vi "YOST 3 Space Loop.vi"() -> ()   [LabVIEW 2012]
uses:
  <vilib>/Platform/TimedLoop/XDataNode/XDataNode.xnode
  <vilib>/Platform/TimedLoop/XDataNode/nitl_modes.ctl
  <vilib>/Platform/TimedLoop/XDataNode/XDNodeRunTimeDep.lvlib
  <vilib>/Platform/TimedLoop/XDataNode/wakeup.ctl
  <vilib>/Platform/TimedLoop/XDataNode/timing_clust.ctl
  YOST 3 Space.lvlib
  <vilib>/robotics/Controls/Compass Indicator/Compass Indicator.xctl
  <vilib>/robotics/Controls/Attitude Indicator/Attitude Indicator.xctl
panel:
  out "LED Mode":i32
  out "IMU Data":T1
  in  "ID Query (True)":bool=TRUE
  out "Attitude Indicator":cluster{"Roll":dbl, "Pitch":dbl}(xcontrol)
  out "Compass Indicator":dbl(xcontrol)
  in  "error in":errorcluster
  out "error out":errorcluster
  in  "stop?":bool
  in  "Debug":bool
  in  "VISA resource name":refnum<visa-resource-name>
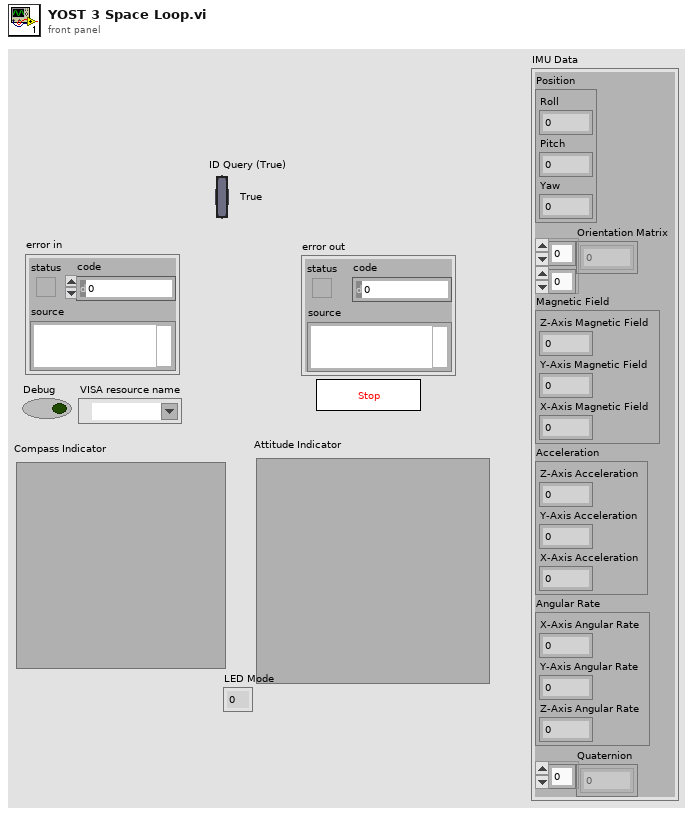
[diagram p1: front panel]
types:
  T1 = cluster{"Position":cluster{"Roll":dbl, "Pitch":dbl, "Yaw":dbl}, "Orientation Matrix":dbl[][], "Magnetic Field":cluster{"Z-Axis Magnetic Field":dbl, "Y-Axis Magnetic Field":dbl, "X-Axis Magnetic Field":dbl}, "Acceleration":cluster{"Z-Axis Acceleration":dbl, "Y-Axis Acceleration":dbl, "X-Axis Acceleration":dbl}, "Angular Rate":cluster{"X-Axis Angular Rate":dbl, "Y-Axis Angular Rate":dbl, "Z-Axis Angular Rate":dbl}, "Quaternion":dbl[]}
  T2 = typedef "XDNodeRunTimeDep.lvlib/timing_clust.ctl" = cluster{"Expected End [f-1]":u64, "Actual End [f-1]":u64, "Finished Late? [f-1]":bool, "Expected End [i-1]":u64, "Actual End [i-1]":u64, "Finished Late? [i-1]":bool, "Expected Start [i]":u64, "Actual Start [i]":u64, "Expected Start [f]":u64, "Actual Start [f]":u64, "Source Name":string, "Structure Name":string, "Period":i64, "Deadline":i64, "Offset":i64, "Start":i64, "Priority":i32, "Timeout":i32, "Mode":T3, "Wakeup Reason":T4, "Error":errorcluster, "Source Type":string, "Secondary Source Type":string, "Global End Time":u64, "Global Start Time":u64, "Frame Duration":u64, "Iteration Duration":u64, "Assigned CPU":i32, "I/O Scan Engine Mode":u32}
  T3 = typedef "XDNodeRunTimeDep.lvlib/nitl_modes.ctl" = enum32{"No Change", "Process missed periods, maintain original phase", "Discard missed periods, maintain original phase", "Process missed periods, ignore original phase", "Discard missed periods, ignore original phase"}
  T4 = typedef "XDNodeRunTimeDep.lvlib/wakeup.ctl" = enum32{"Normal", "Aborted", "Asynchronous wakeup", "Timing source error", "Timed loop error", "Timeout"}
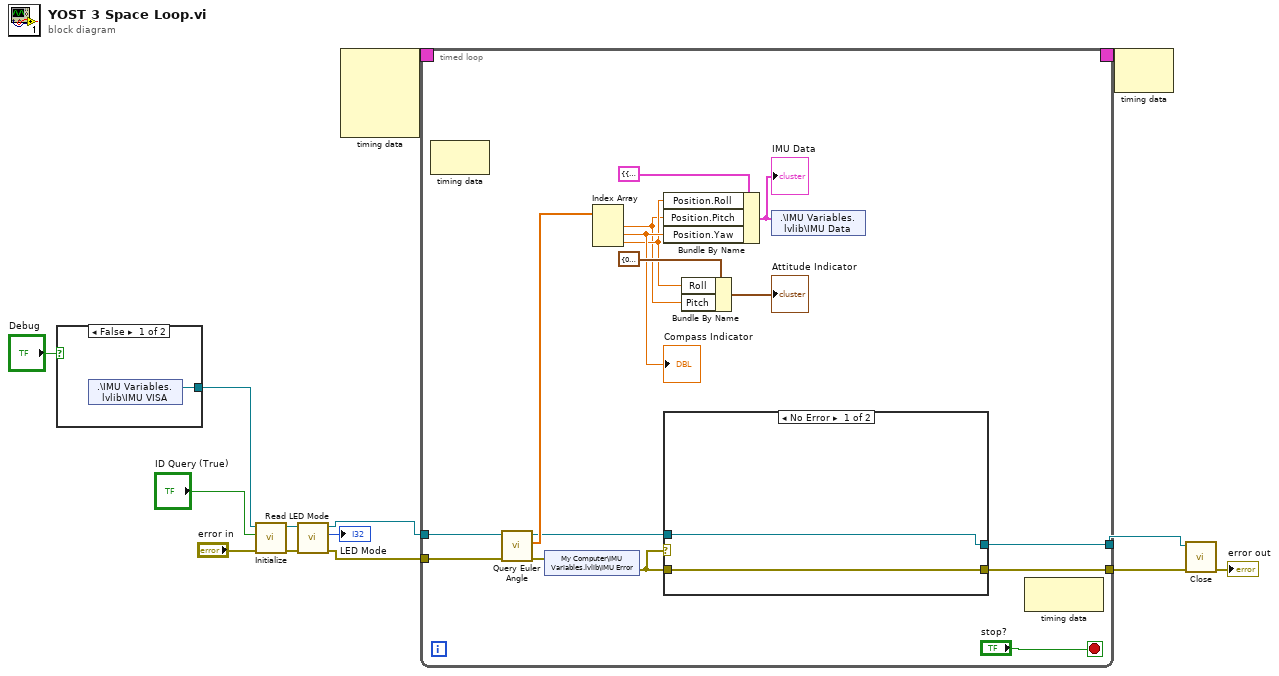
[diagram p0: block diagram]
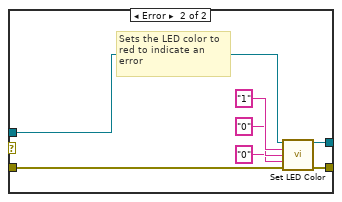
[diagram p2: hidden frame]
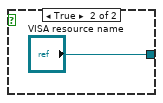
[diagram p3: hidden frame]
diagram:
  n1 = case shown="False" "Debug" {
    tunnel: [w15 "VISA resource name"] -> w10
    frame False {
      n2 = shared-variable ".\\IMU Variables.lvlib\\IMU VISA"() -> (w15:refnum<visa-resource-name>)  [unwired: 1 in, 1 out]
    }
    frame True {
    }
  }
  n3 = call "Initialize.vi"("error in (no error)"="error in", "ID Query (True)"="ID Query (True)", "VISA resource name"=w10) -> ("error out"=w6:errorcluster, "VISA resource name out"=w5:refnum<visa-resource-name>)  [unwired: 7 in]
  n4 = call "Read LED Mode.vi"("error in"=w6, "Session In"=w5) -> ("error out"=w7:errorcluster, "Mode"=→"LED Mode":i32, "Session Out"=w4:refnum<visa-resource-name>)  [unwired: 7 in]
  n5 = node-c288() -> (w13:T2)  [unwired: 4 in]
  n6 = timed-loop {
    timing: w13 -> [_]
    timing-out: [_] -> w12
    tunnel: [w17] -> w1
    tunnel: w4 -> [w22]
    tunnel: w7 -> [w21]
    tunnel: [w18] -> w2
    stop <- "stop?" stop-if-true
    n7 = node-c288() -> ()  [unwired: 1 in, 1 out]
    n8 = call "Query Euler Angle.vi"("error in"=w21, "Session In"=w22) -> ("error out"=w20:errorcluster, "Euler Angles"=w29:dbl[], "Session Out"=w19:refnum<visa-resource-name>)  [unwired: 7 in]
    n9 = shared-variable "My Computer\\IMU Variables.lvlib\\IMU Error"(w20) -> (error out=w23:errorcluster)  [unwired: 1 in]
    n10 = Index Array(array=w29) -> (element #1=w24:dbl, element #2=w26:dbl, element #3=w25:dbl)  [unwired: 3 in]
    "Compass Indicator" <- w26
    n11 = Bundle By Name(cluster=T1 {"Position"={"Roll"=0.0, "Pitch"=0.0, "Yaw"=0.0}, "Orientation Matrix"=[], "Magnetic Field"={"Z-Axis Magnetic Field"=0.0, "Y-Axis Magnetic Field"=0.0, "X-Axis Magnetic Field"=0.0}, "Acceleration"={"Z-Axis Acceleration"=0.0, "Y-Axis Acceleration"=0.0, "X-Axis Acceleration"=0.0}, "Angular Rate"={"X-Axis Angular Rate"=0.0, "Y-Axis Angular Rate"=0.0, "Z-Axis Angular Rate"=0.0}, "Quaternion"=[]} ("IMU Data"), "Position.Roll"=w25, "Position.Pitch"=w24, "Position.Yaw"=w26) -> (w31:T1)
    "IMU Data" <- w31
    n12 = case shown="No Error" w23 {
      tunnel: [w33 w41] -> w17
      tunnel: [w34 w40] -> w18
      tunnel: w23 -> [w34 w39]
      tunnel: w19 -> [w33 w35]
      frame No Error {
      }
      frame Error {
        # "Sets the LED color to red to indicate an error"
        n13 = call "Set LED Color.vi"("Session In"=w35, "Red"="1", "Blue"="0", "Green"="0", "error in"=w39) -> ("Session Out"=w41:refnum<visa-resource-name>, "error out"=w40:errorcluster)  [unwired: 9 in]
      }
    }
    n14 = Bundle By Name(cluster=cluster{"Roll":dbl, "Pitch":dbl} {"Roll"=0.0, "Pitch"=0.0} ("Attitude Indicator"), "Roll"=w25, "Pitch"=w24) -> (→"Attitude Indicator":cluster{"Roll":dbl, "Pitch":dbl})
    n15 = shared-variable ".\\IMU Variables.lvlib\\IMU Data"(w31) -> ()  [unwired: 1 in, 1 out]
    n16 = node-c288() -> ()  [unwired: 1 in, 1 out]
  }
  n17 = node-c288(w12) -> ()  [unwired: 1 out]
  n18 = call "Close.vi"("error in (no error)"=w2, "VISA resource name"=w1) -> ("error out"=→"error out":errorcluster)  [unwired: 9 in]
